vi "Task Factory.vi"(11 "Task Ref":refnum<class "Build_Javier_Lopez_lib_Configuration_Filejson class.lvclass">) -> (0 "error out":errorcluster, 2 "Item Names":string[](array[string]))   [LabVIEW 2021, in "Task Base.lvclass"]
uses:
  Task Base.lvclass
  <vilib>/Javier Lopez/Configuration File/Json Element/Build_Javier_Lopez_lib_Configuration_Filejson class.lvclass
  Module Launcher Base/Launcher Base.lvclass
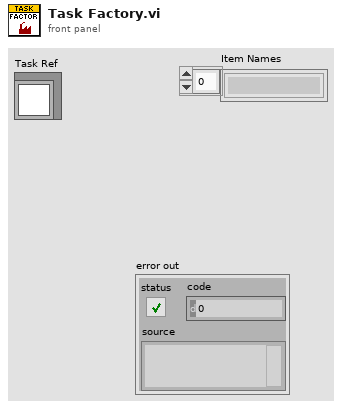
[diagram p1: front panel]
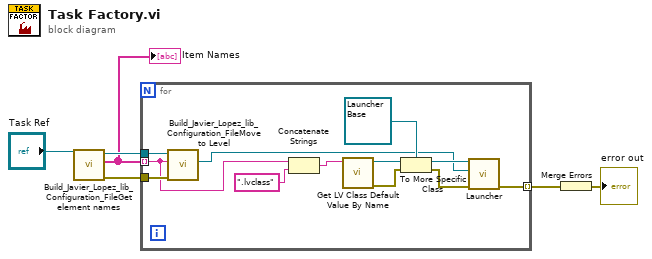
[diagram p0: block diagram]
diagram:
  n1 = call-dynamic "Build_Javier_Lopez_lib_Configuration_FileGet element names.vi"("json class in"="Task Ref") -> ("error out"=w2:errorcluster, "Item Names"=w1:string[], "json class out"=w5:refnum<class "Build_Javier_Lopez_lib_Configuration_Filejson class.lvclass">)  [unwired: 8 in]
  "Item Names" <- w1
  n2 = for {
    tunnel: w1 -> [w7] mode=indexing
    tunnel: w5 -> [w10]
    tunnel: [w11] -> w4 mode=indexing
    tunnel: w2 -> [w9]
    n3 = call-dynamic "Build_Javier_Lopez_lib_Configuration_FileMove to Level.vi"("error in (no error)"=w9, "Element"=w7, "json class in"=w10) -> ("New json class"=w8:refnum<class "Build_Javier_Lopez_lib_Configuration_Filejson class.lvclass">)  [unwired: 6 in, 2 out]
    n4 = Concatenate Strings(w7, ".lvclass" ("string")) -> (w18:string)
    n5 = call <vilib>:"Get LV Class Default Value By Name.vi"("class name"=w18) -> ("error out"=w15:errorcluster, "object"=w14:refnum<class>)  [unwired: 9 in]
    n6 = To More Specific Class(target class=refnum<class "Launcher Base.lvclass"> refnum ("Module Launcher Base"), reference=w14, error in=w15) -> (specific class reference=w16:refnum<class "Launcher Base.lvclass">, error out=w17:errorcluster)
    n7 = call-dynamic "Launcher.vi"("error in (no error)"=w17, "Log Class"=w8, "Module Launcher Base in"=w16) -> ("error out"=w11:errorcluster)  [unwired: 8 in]
  }
  n8 = Merge Errors(w4) -> (→"error out":errorcluster)
